vi "Day 05 Part 2.vi"(11 "Input":string) -> (3 "Output":u32)   [LabVIEW 2021]
panel:
  out "Intensity Graph":i32[][](graph)
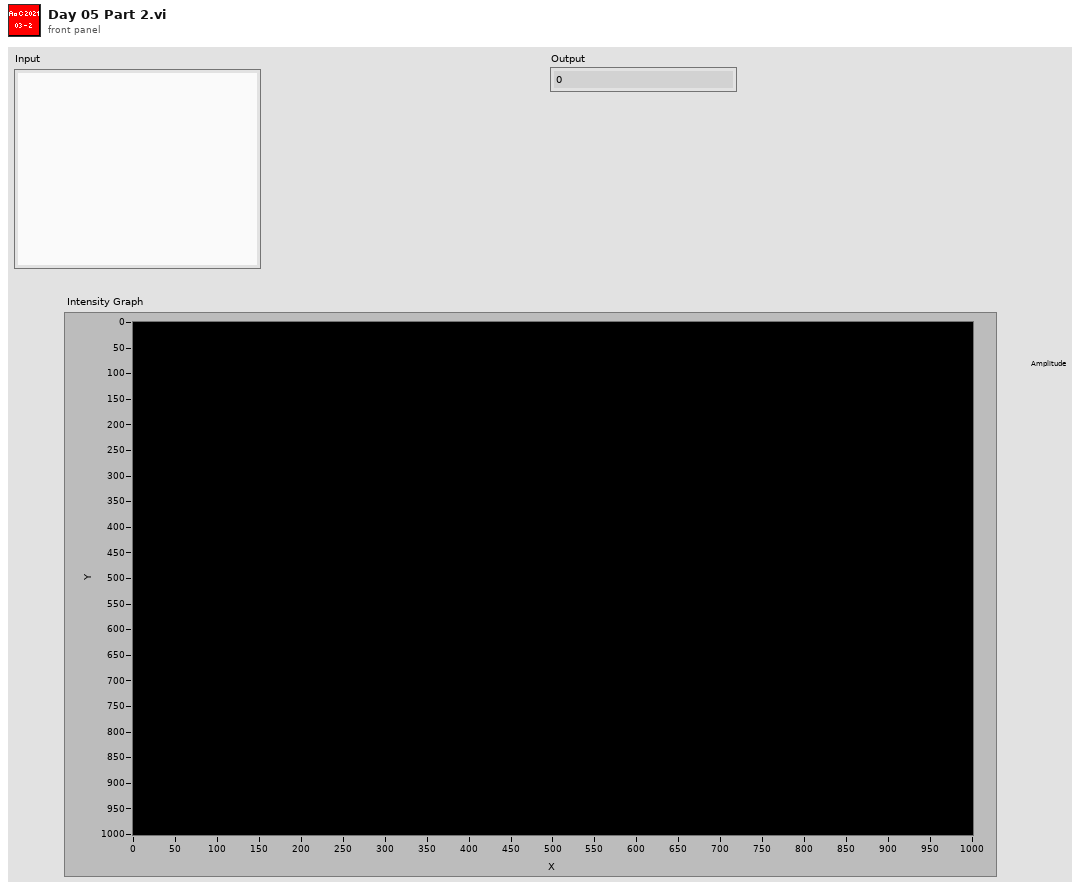
[diagram p1: front panel]
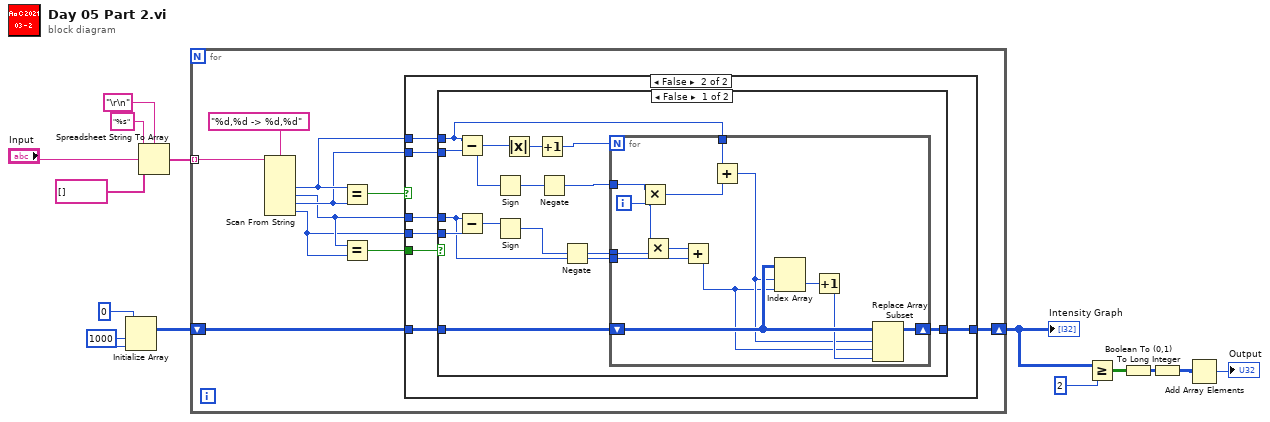
[diagram p0: block diagram]
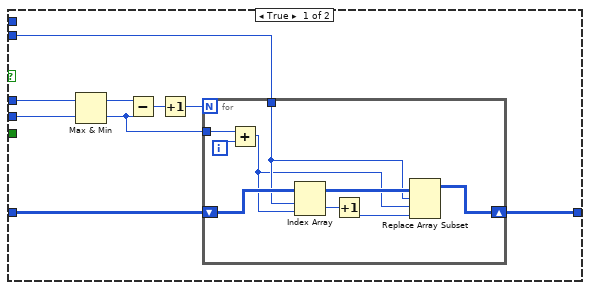
[diagram p2: hidden frame]
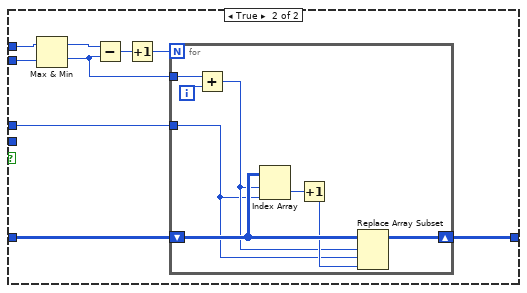
[diagram p3: hidden frame]
diagram:
  w10 = 1000 ("dimension size")
  n1 = Initialize Array(0, w10, w10) -> (w5:i32[][])
  n2 = Spreadsheet String To Array(delimiter (Tab)="\r\n", format string="%s", spreadsheet string="Input", array type (2D Dbl)=string[] []) -> (array=w11:string[])
  n3 = for {
    tunnel: w11 -> [w24] mode=indexing
    shift-right: [w15] -> w4
    shift-left: w5 -> [w16]
    n4 = Scan From String(format string="%d,%d -> %d,%d", input string=w24) -> (output 1=w22:i32, output 2=w20:i32, output 3=w21:i32, output 4=w19:i32)  [unwired: 6 in, 3 out]
    n5 = Equal?(x=w22, y=w21) -> (x = y?=w18:bool)
    n6 = Equal?(x=w20, y=w19) -> (x = y?=w17:bool)
    n7 = case shown="False" w18 {
      tunnel: w22 -> [_ w48]
      tunnel: w21 -> [w31 w47]
      tunnel: w20 -> [w30 w46]
      tunnel: w19 -> [w29 w42]
      tunnel: w17 -> [_ w45]
      tunnel: w16 -> [w26 w44]
      tunnel: [w25 w43] -> w15
      frame True {
        n8 = Max & Min(x=w30, y=w29) -> (max(x,y)=w28:i32, min(x,y)=w27:i32)
        n9 = Subtract(x=w28, y=w27) -> (x-y=w33:i32)
        n10 = Increment(x=w33) -> (x+1=w32:i32)
        n11 = for {
          N: w32 -> [_]
          tunnel: w27 -> [w40]
          tunnel: w31 -> [w36]
          shift-right: [w34] -> w25
          shift-left: w26 -> [w38]
          i -> [w41]
          n12 = Add(x=w40, y=w41) -> (x+y=w35:i32)
          n13 = Index Array(array=w38, index (row)=w36, index (col)=w35) -> (element=w39:i32)
          n14 = Increment(x=w39) -> (x+1=w37:i32)
          n15 = Replace Array Subset(array=w38, new element=w37, index (row)=w36, index (col)=w35) -> (w34:i32[][])
        }
      }
      frame False {
        n16 = case shown="False" w45 {
          tunnel: w48 -> [w56 w82]
          tunnel: w47 -> [w62 w80]
          tunnel: w46 -> [w55 w78]
          tunnel: w44 -> [w58 w77]
          tunnel: [w57 w76] -> w43
          tunnel: w42 -> [w61 _]
          frame False {
            n17 = Subtract(x=w56, y=w62) -> (x-y=w54:i32)
            n18 = Subtract(x=w55, y=w61) -> (x-y=w52:i32)
            n19 = Sign(1:w54) -> (0:w53:i32)
            n20 = Sign(1:w52) -> (0:w51:i32)
            n21 = Absolute Value(x=w54) -> (abs(x)=w60:i32)
            n22 = Increment(x=w60) -> (x+1=w59:i32)
            n23 = Negate(x=w53) -> (-x=w50:i32)
            n24 = Negate(x=w51) -> (-x=w49:i32)
            n25 = for {
              N: w59 -> [_]
              shift-right: [w71] -> w57
              shift-left: w58 -> [w74]
              tunnel: w50 -> [w70]
              tunnel: w49 -> [w67]
              tunnel: w56 -> [w66]
              tunnel: w55 -> [w64]
              i -> [w68]
              n26 = Multiply(x=w70, y=w68) -> (x*y=w69:i32)
              n27 = Multiply(x=w68, y=w67) -> (x*y=w65:i32)
              n28 = Add(x=w65, y=w64) -> (x+y=w63:i32)
              n29 = Add(x=w66, y=w69) -> (x+y=w72:i32)
              n30 = Index Array(array=w74, index (row)=w72, index (col)=w63) -> (element=w75:i32)
              n31 = Increment(x=w75) -> (x+1=w73:i32)
              n32 = Replace Array Subset(array=w74, new element=w73, index (row)=w72, index (col)=w63) -> (w71:i32[][])
            }
          }
          frame True {
            n33 = Max & Min(x=w82, y=w80) -> (max(x,y)=w81:i32, min(x,y)=w79:i32)
            n34 = Subtract(x=w81, y=w79) -> (x-y=w84:i32)
            n35 = Increment(x=w84) -> (x+1=w83:i32)
            n36 = for {
              N: w83 -> [_]
              tunnel: w79 -> [w91]
              tunnel: w78 -> [w86]
              shift-right: [w85] -> w76
              shift-left: w77 -> [w89]
              i -> [w92]
              n37 = Add(x=w91, y=w92) -> (x+y=w87:i32)
              n38 = Index Array(array=w89, index (row)=w87, index (col)=w86) -> (element=w90:i32)
              n39 = Increment(x=w90) -> (x+1=w88:i32)
              n40 = Replace Array Subset(array=w89, new element=w88, index (row)=w87, index (col)=w86) -> (w85:i32[][])
            }
          }
        }
      }
    }
  }
  "Intensity Graph" <- w4
  n41 = Greater Or Equal?(x=w4, y=2) -> (x >= y?=w7:bool[][])
  n42 = Boolean To (0,1)(Boolean=w7) -> (0, 1=w6:i16[][])
  n43 = To Long Integer(number=w6) -> (32bit integer=w3:i32[][])
  n44 = Add Array Elements(numeric array=w3) -> (sum=→"Output":i32)
